vi "File Writing.vi"() -> (0 "new file path (Not A Path if cancelled)":path)   [LabVIEW 2014]
uses:
  <vilib>/Utility/file.llb/Write To Spreadsheet File (DBL).vi
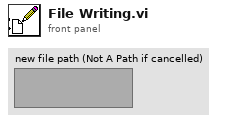
[diagram p1: front panel]
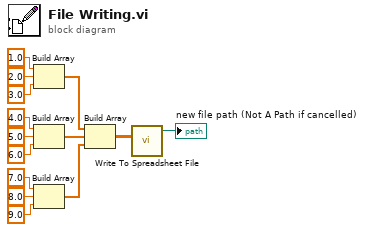
[diagram p0: block diagram]
diagram:
  n1 = Build Array(1.0 ("element"), 2.0 ("element"), 3.0 ("element")) -> (w5:dbl[])
  n2 = Build Array(4.0 ("element"), 5.0 ("element"), 6.0 ("element")) -> (w4:dbl[])
  n3 = Build Array(7.0 ("element"), 8.0 ("element"), 9.0 ("element")) -> (w3:dbl[])
  n4 = Build Array(w5, w4, w3) -> (w2:dbl[][])
  n5 = call-poly <vilib>:"Write To Spreadsheet File.vi"("2D data"=w2) -> ("new file path (Not A Path if cancelled)"=→"new file path (Not A Path if cancelled)":path)  [unwired: 7 in]
